vi "te_20200903.vi"() -> ()   [LabVIEW 2018]
uses:
  TE_ControlType_Enum.ctl
  TE_Polarity_Enum.ctl
  te_state.ctl
  TE_Main_Clust.ctl
  TE_Serial_Config_Clust.ctl
  Epimedia_Connex_Source/Controls/Clusts/TE_Data_Clust.ctl
  Epimedia_Connex_Source/Controls/Enums/WatchdogTimer_Enum.ctl
  Epimedia_Connex_Source/Controls/Enums/LogLoopEnum.ctl
  Disdrometer/UserConfig_ChannelSettings_Clust.ctl
panel:
  out "Shutdown if Alarm 3":bool
  out "Shutdown if Alarm 2":bool
  out "Shutdown if Alarm":bool
  out "LoAlarm3":dbl format="%.2g"
  out "LoAlarm2":dbl format="%.2g"
  out "LoAlarm":dbl format="%.2g"
  out "HiAlarm3":dbl format="%.2g"
  out "HiAlarm2":dbl format="%.2g"
  out "HiAlarm":dbl format="%.2g"
  out "Alarms? 3":bool
  out "Alarms? 2":bool
  out "Alarms?":bool
  in  "Shutdown if Alarm":bool=TRUE
  in  "Low Alarm":dbl=30.0 format="%.2g"
  in  "High Alarm":dbl=50.0 format="%.2g"
  in  "Alarms?":bool=TRUE
  out "AlarmStatus 3":T1(ring)
  out "AlarmStatus 2":T1(ring)
  out "AlarmStatus":T1(ring)
  out "On? 3":bool
  out "On? 2":bool
  in  "WriteFront":bool
  in  "WriteBottom":bool
  out "Polarity 3":T2
  out "Control Type 3":T3
  out "P 3":dbl format="%.2g"
  out "I 3":dbl format="%.2g"
  out "D 3":dbl format="%.2g"
  out "Set Point 3":dbl format="%.2g"
  out "Temp 3":dbl format="%.2g"
  out "Output 3":dbl format="%.2f"
  out "Polarity 2":T2
  out "Control Type 2":T3
  out "P 2":dbl format="%.2g"
  out "I 2":dbl format="%.2g"
  out "D 2":dbl format="%.2g"
  out "Set Point 2":dbl format="%.2g"
  out "Temp 2":dbl format="%.2g"
  out "Output 2":dbl format="%.2f"
  out "Polarity 4":T2
  in  "Polarity":T2 caption="Polarity*"
  out "Control Type 4":T3
  in  "Control Type":T3=enum."PID"
  in  "WriteAir":bool
  out "status":bool
  out "code":i32
  out "Read Progress":dbl(slide) scale=0.0..1.0
  out "On?":bool
  out "P 4":dbl format="%.2g"
  out "I 4":dbl format="%.2g"
  out "D 4":dbl format="%.2g"
  out "Set Point 4":dbl format="%.2g"
  out "Temp":dbl format="%.2g"
  out "Output":dbl format="%.2f"
  in  "On?":bool=TRUE
  in  "P":dbl=5.0 format="%.2g"
  in  "I":dbl format="%.2g"
  in  "D":dbl format="%.2g"
  in  "Set Point":dbl=40.0 format="%.2g"
  out "Header":picture
  in  "Address":string[](array[string])=["01", "02", "03"]
  in  "Port":refnum<visa-resource-name>="Port1"
  in  "stop":bool
  out "Error Dialog":string="Error Message Display Box"
  out "Waveform Chart":cluster{"[0]":dbl, "[0]":dbl, "[0]":dbl}(graph)
  # "°C"
  # "Temp."
  # "%"
  # "Output"
  # "°C"
  # "*Normal Polarity is WP1+ and WP2-\n  Reverse polarity is WP2+ and WP1-"
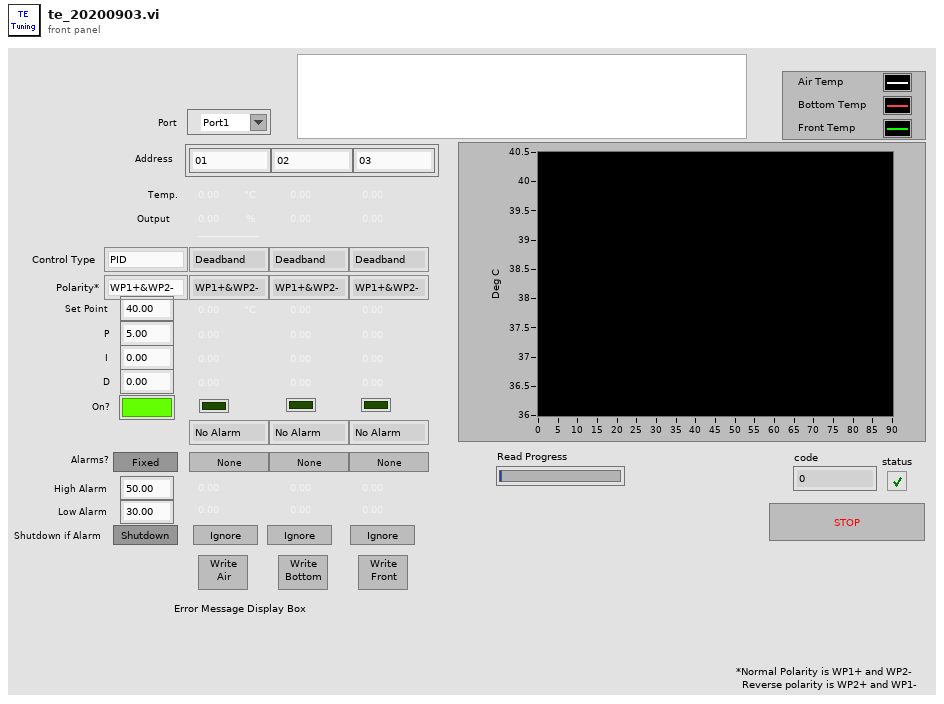
[diagram p1: front panel]
types:
  T1 = enum16{"No Alarm", "High Alarm", "Low Alarm", "Both Alarms"}
  T2 = typedef "TE_Polarity_Enum.ctl" = enum16{"WP1+&WP2-", "WP2+&WP1-"}
  T3 = typedef "TE_ControlType_Enum.ctl" = enum16{"Deadband", "PID", "Computer"}
  T4 = typedef "TE_Main_Clust.ctl" = cluster{"Serial":T5, "AcqData":dbl[][], "AcqSorted":T6, "WriteChannel":i32, "ErrMsg":string}
  T5 = typedef "TE_Serial_Config_Clust.ctl" = cluster{"port":refnum<visa-resource-name>, "timeout":u32, "baud":u32, "dataBits":u16, "stopBits":u16, "flowControl":u16, "parity":u16, "termChar":bool, "checkSum":bool, "checkSumVal":string, "Address":string[]}
  T6 = typedef "TE_Data_Clust.ctl" = cluster{"TimeString":string, "TimeStamp":dbl, "Temp":dbl, "Output":dbl, "Temp 2":dbl, "Output 2":dbl, "Temp 3":dbl, "Output 3":dbl}
  T7 = typedef "te_state.ctl" = enum16{"TE_Init", "TE_Autotune", "TE_Wait", "TE_Read", "TE_Display", "TE_Send", "TE_Write"}
  T8 = typedef "WatchdogTimer_Enum.ctl" = enum16{"ResetAll", "CheckAll", "HW1", "HW2", "Tones", "FP", "Noise", "Log", "TCP", "AI", "TC", "ADAM", "Disdrom", "TE", "Weather"}
  T9 = typedef "LogLoopEnum.ctl" = enum16{"Log_Init", "Log_Config", "Log_CfgAlarm", "Log_TimeDomain", "Log_Tone", "Log_NoiseTrace", "Log_NoiseSum", "Log_DO", "Log_AI", "Log_TC", "Log_Disdrom", "Log_Weather", "Log_TE", "Log_ADAM", "Log_UPS", "Log_ChkTime", "Log_Alarm", "Log_SSH", "Log_Write", "Log_Exit"}
  T10 = typedef "UserConfig_ChannelSettings_Clust.ctl" = cluster{"Set Point":dbl, "Control Type":T3, "Polarity":T2, "P":dbl, "I":dbl, "D":dbl, "On?":bool, "Alarms?":bool, "High Alarm":dbl, "Low Alarm":dbl, "Shutdown if Alarm":bool}
  T11 = typedef "imagedata.ctl" = cluster{"image type":i32, "image depth":i32, "image":u8[], "mask":u8[], "colors":u32[], "Rectangle":cluster{"left":i16, "top":i16, "right":i16, "bottom":i16}}
  T12 = cluster{"AcqData[0]":dbl, "AcqData[1]":dbl, "AcqData[2]":dbl, "AcqData[3]":dbl, "AcqData[4]":dbl, "AcqData[5]":dbl, "AcqData[6]":dbl, "AcqData[7]":dbl, "AcqData[8]":dbl, "AcqData[9]":dbl, "AcqData[10]":dbl, "AcqData[11]":dbl, "AcqData[12]":dbl, "AcqData[13]":dbl}
  T13 = cluster{"AcqData[0]":dbl, "AcqData[0]":dbl, "AcqData[0]":dbl}
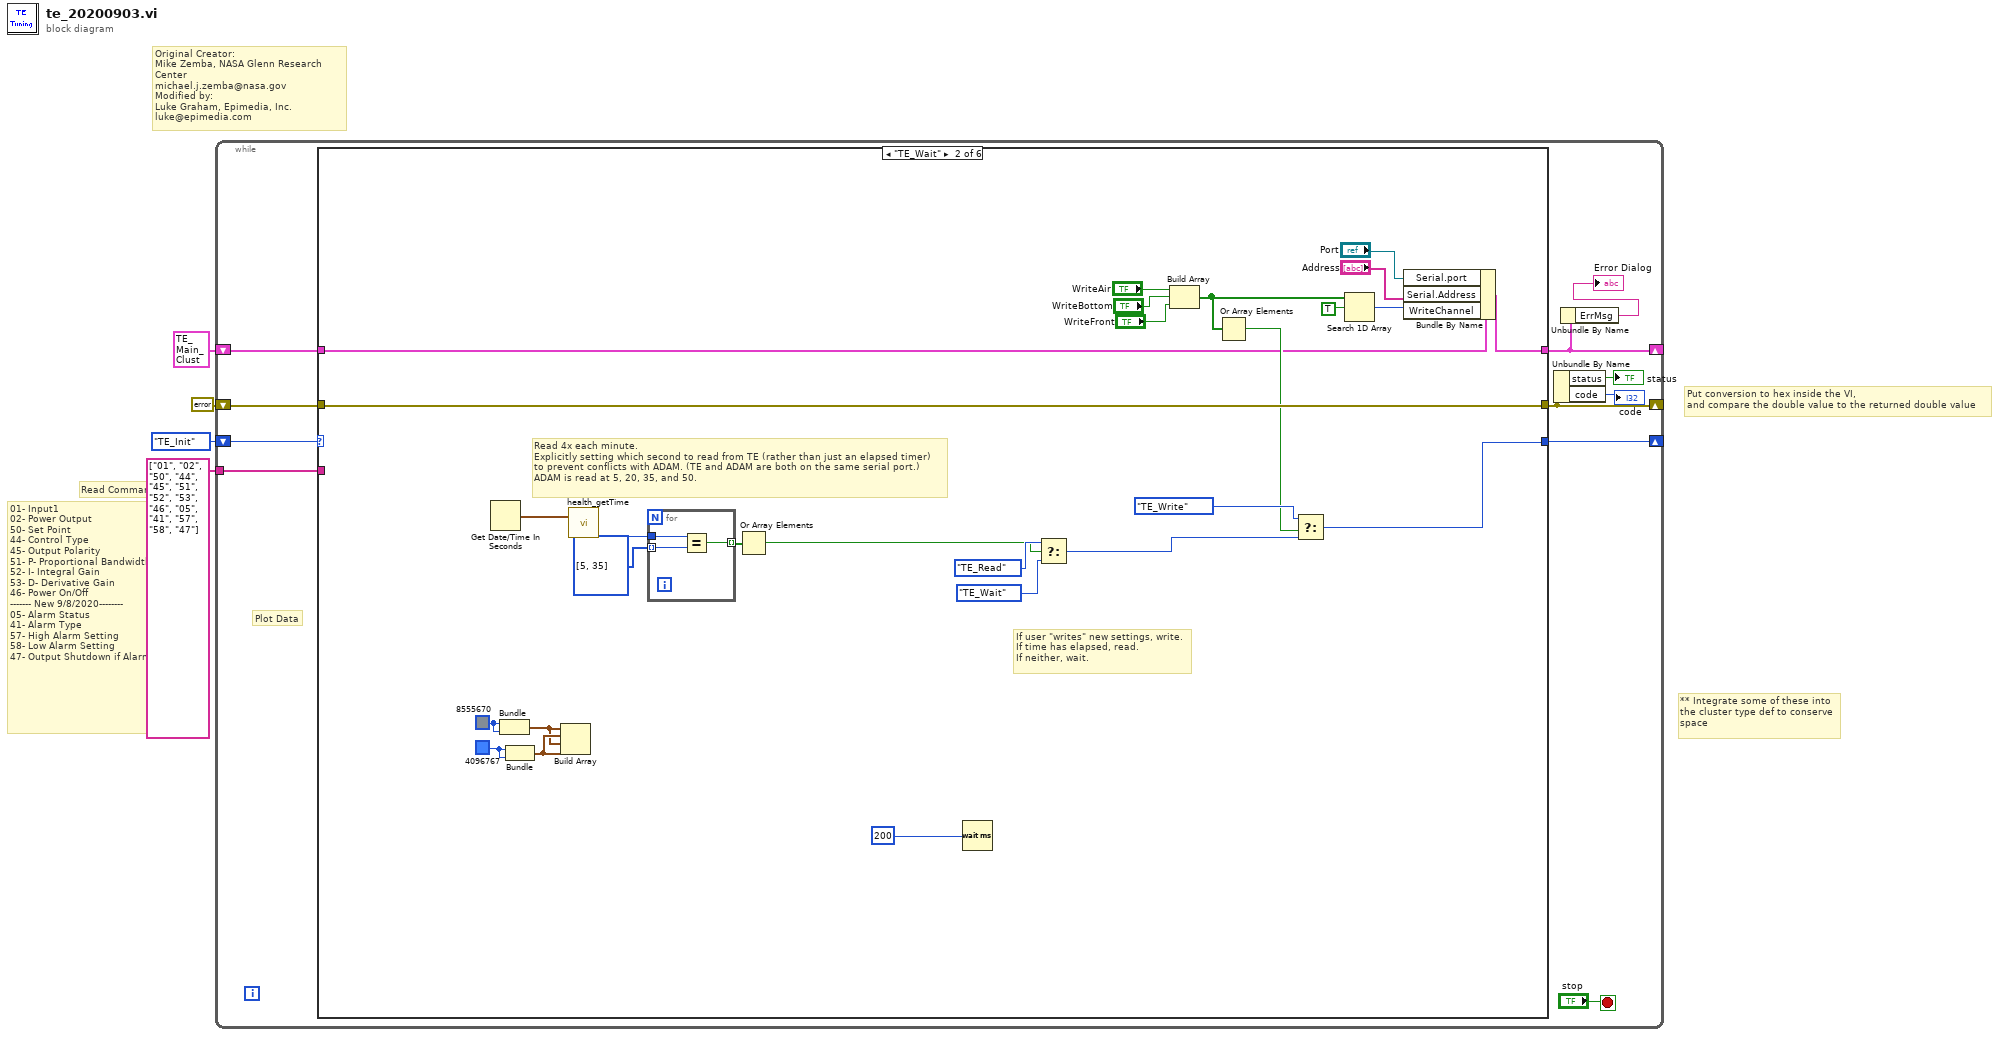
[diagram p0: block diagram]
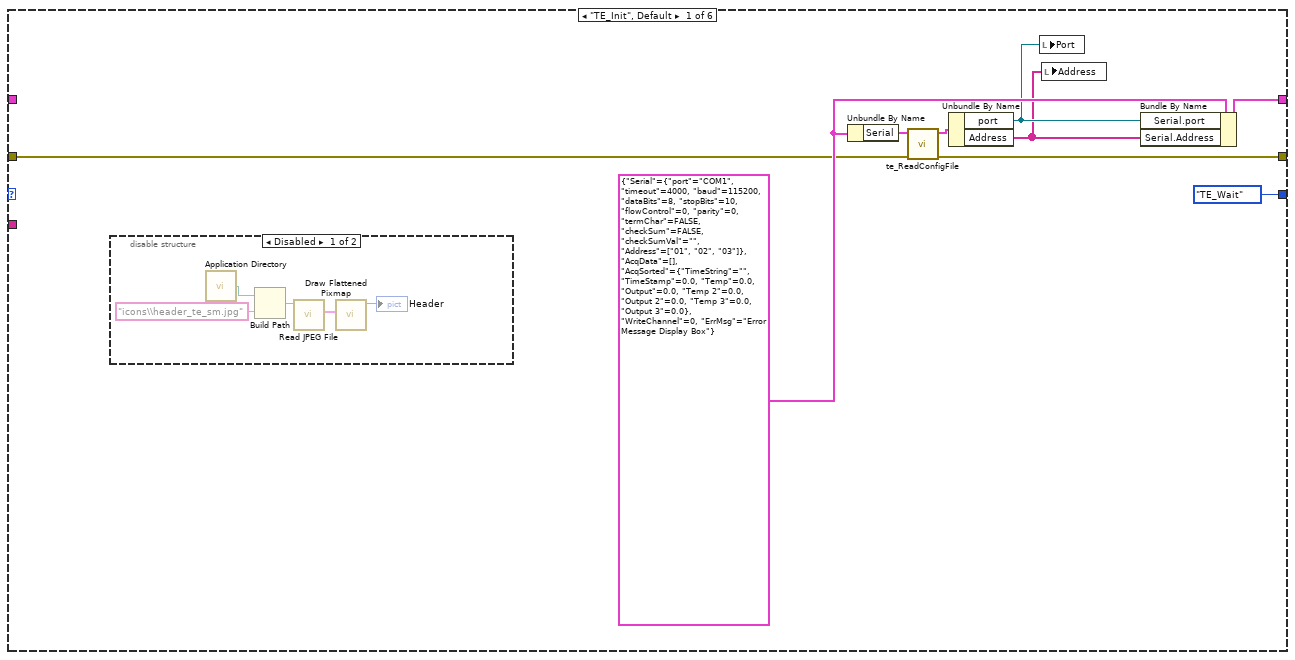
[diagram p2: hidden frame]
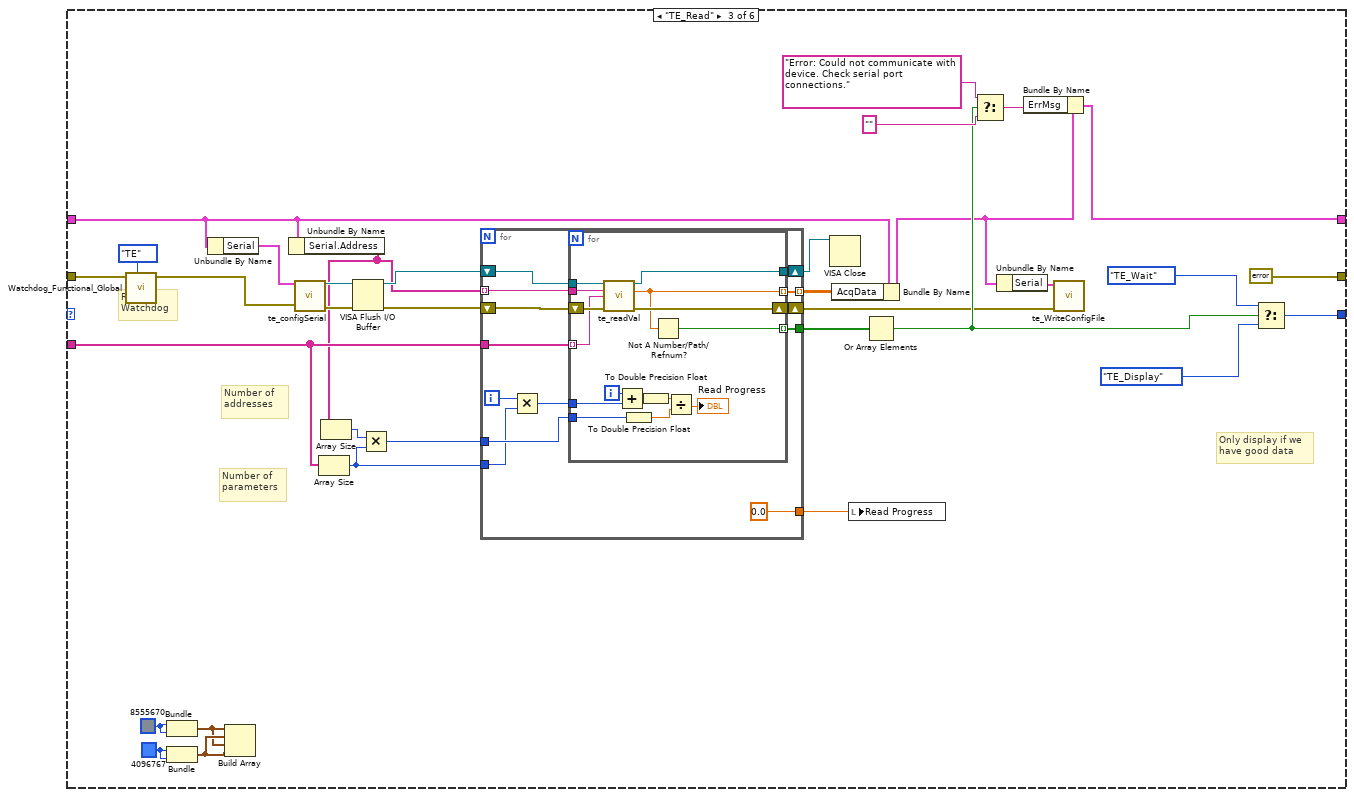
[diagram p4: hidden frame]
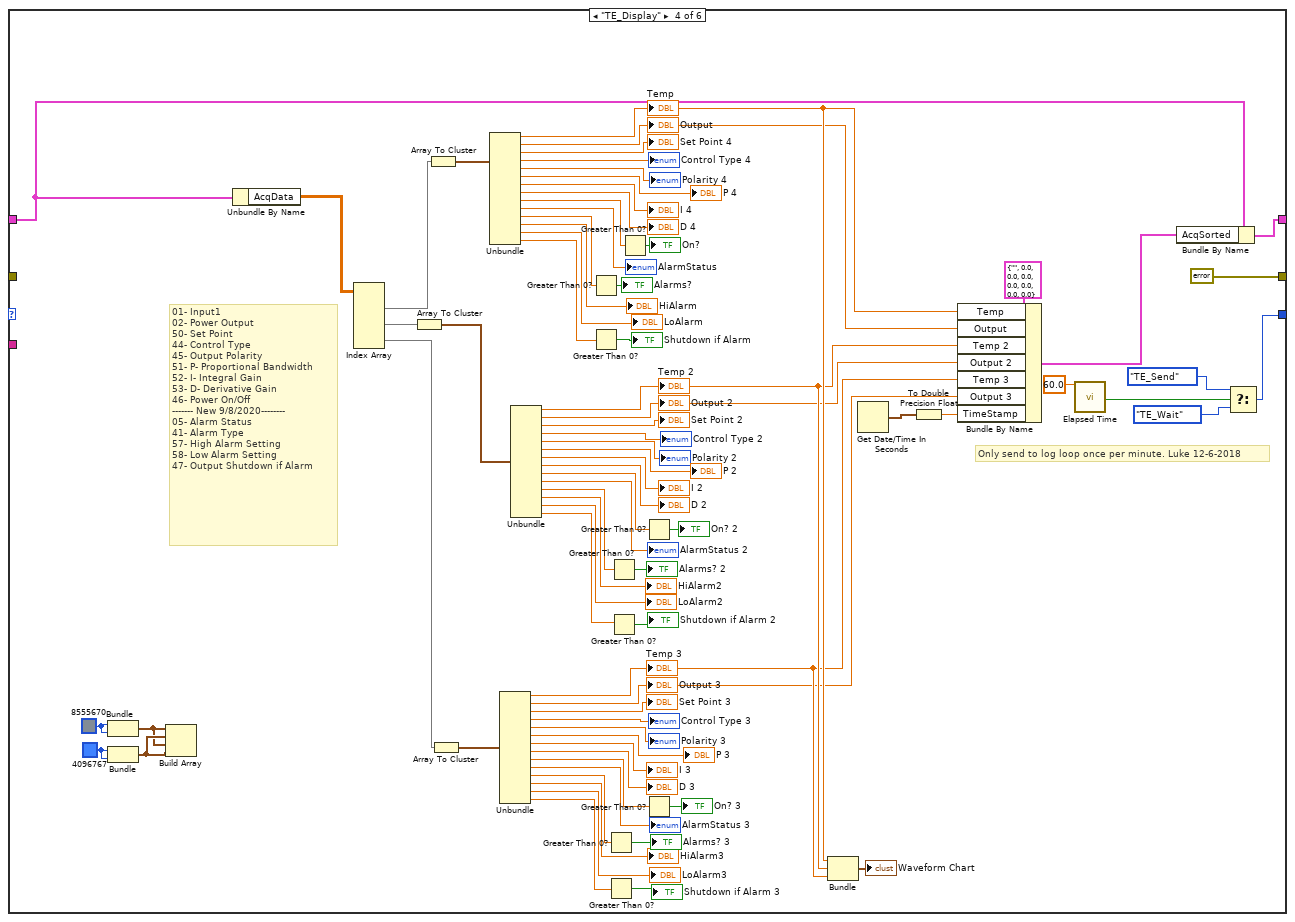
[diagram p5: hidden frame]
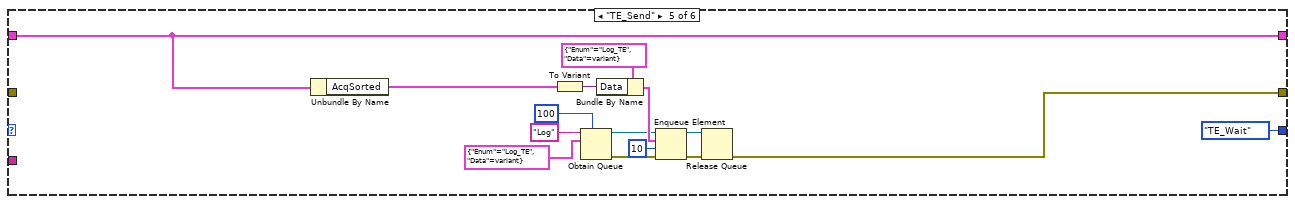
[diagram p6: hidden frame]
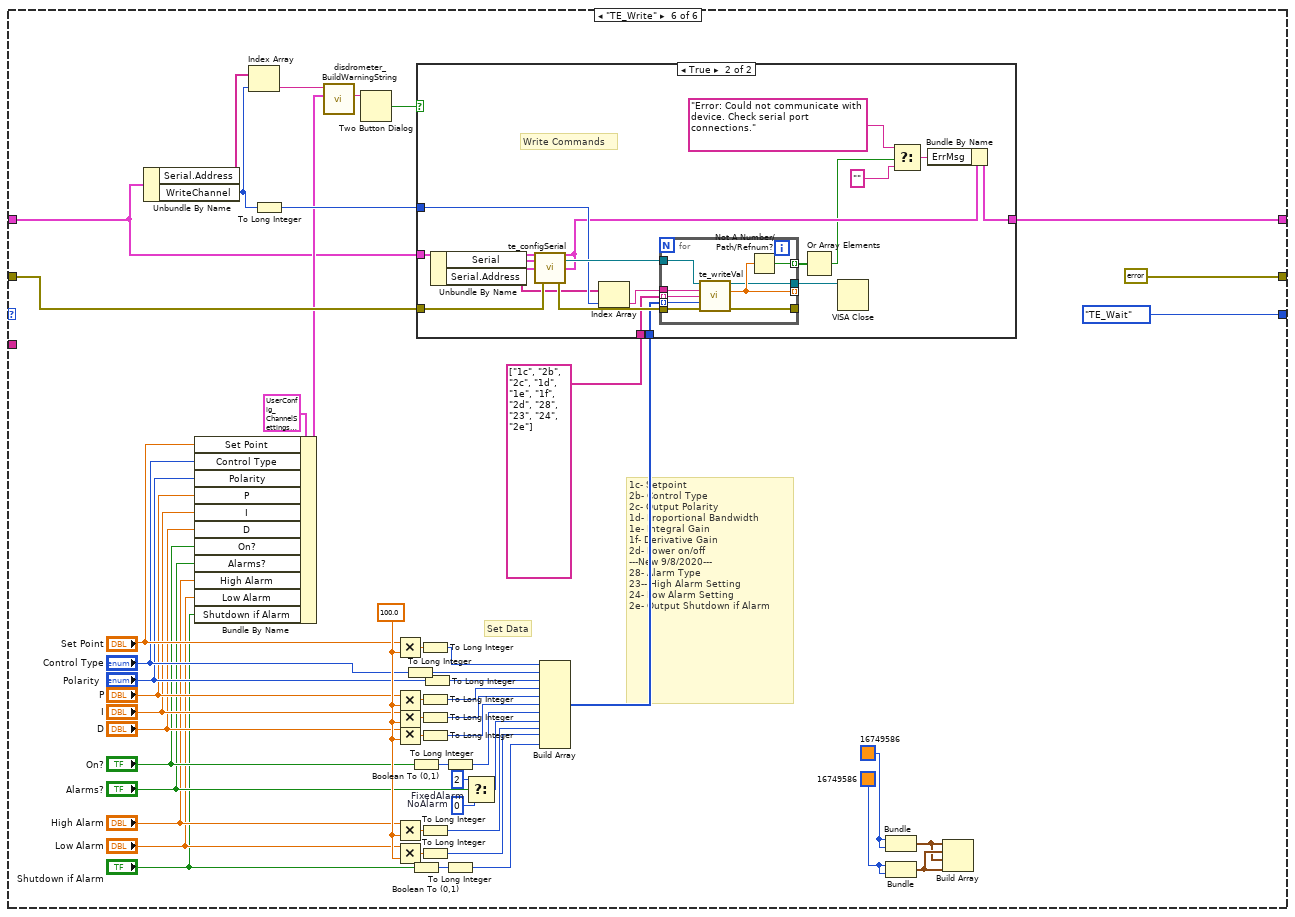
[diagram p7: hidden frame]
diagram:
  # "Original Creator: \nMike Zemba, NASA Glenn Research Center\nmichael.j.zemba@nasa.gov\nModified by:\nLuke Graham, Epimedia, Inc.\nluke@epimedia.com"
  # "Put conversion to hex inside the VI,\nand compare the double value to the returned double value"
  # "Read Commands"
  # "01- Input1\n02- Power Output\n50- Set Point\n44- Control Type\n45- Output Polarity\n51- P- Proportional Bandwidth\n52- I- Integral Gain\n53- D- Derivative Gain\n46- Power On/Off\n------- New 9/8/2020--------\n05- Alarm Status\n41- Alarm Type\n57- High Alarm Setting\n58- Low Alarm Setting\n47- Output Shutdown if Alarm"
  # "** Integrate some of these into\nthe cluster type def to conserve\nspace"
  n1 = while {
    shift-right: [w14] -> _
    shift-left: te_state."TE_Init" ("Enum") -> [w15]
    shift-right: [w9] -> _
    shift-left: errorcluster {"status"=FALSE, "code"=0, "source"=""} ("Error Out") -> [w13]
    tunnel: string[] ["01", "02", "50", "44", "45", "51", "52", "53", "46", "05", "41", "57", "58", "47"] -> [w10]
    shift-right: [w6] -> _
    shift-left: T4 {"Serial"={"port"="COM1", "timeout"=4000, "baud"=115200, "dataBits"=8, "stopBits"=10, "flowControl"=0, "parity"=0, "termChar"=FALSE, "checkSum"=FALSE, "checkSumVal"="", "Address"=["01", "02", "03"]}, "AcqData"=[], "AcqSorted"={"TimeString"="", "TimeStamp"=0.0, "Temp"=0.0, "Output"=0.0, "Temp 2"=0.0, "Output 2"=0.0, "Temp 3"=0.0, "Output 3"=0.0}, "WriteChannel"=0, "ErrMsg"="Error Message Display Box"} -> [w11]
    stop <- "stop" stop-if-true
    # "Plot Data"
    n2 = case shown="\"TE_Wait\"" w15 {
      tunnel: [te_state."TE_Wait" ("Enum") w46 w72 w161 te_state."TE_Wait" ("Enum") te_state."TE_Wait" ("Enum")] -> w14
      tunnel: w13 -> [w20 w52 w61 _ _ w257]
      tunnel: [w21 w52 errorcluster {"status"=FALSE, "code"=0, "source"=""} ("Error Out") errorcluster {"status"=FALSE, "code"=0, "source"=""} ("Error Out") w197 errorcluster {"status"=FALSE, "code"=0, "source"=""} ("Error Out")] -> w9
      tunnel: w11 -> [_ w33 w74 w164 w207 w217]
      tunnel: w10 -> [_ _ w82 _ _ _]
      tunnel: [w19 w34 w68 w165 w207 w218] -> w6
      frame "TE_Init", Default {
        w23 = T4 {"Serial"={"port"="COM1", "timeout"=4000, "baud"=115200, "dataBits"=8, "stopBits"=10, "flowControl"=0, "parity"=0, "termChar"=FALSE, "checkSum"=FALSE, "checkSumVal"="", "Address"=["01", "02", "03"]}, "AcqData"=[], "AcqSorted"={"TimeString"="", "TimeStamp"=0.0, "Temp"=0.0, "Output"=0.0, "Temp 2"=0.0, "Output 2"=0.0, "Temp 3"=0.0, "Output 3"=0.0}, "WriteChannel"=0, "ErrMsg"="Error Message Display Box"}
        n3 = disable-structure shown="Disabled" {
          frame Disabled {
            n4 = call <vilib>:"Application Directory.vi"() -> ("Application Directory"=w26:path)
            n5 = Build Path(base path=w26, name or relative path="icons\\header_te_sm.jpg") -> (appended path=w27:path)
            n6 = call <vilib>:"Read JPEG File.vi"("path to JPEG file"=w27) -> ("image data"=w29:T11)  [unwired: 8 in, 2 out]
            n7 = call <vilib>:"Draw Flattened Pixmap.vi"("image data"=w29) -> ("new picture"=→"Header":picture)  [unwired: 8 in]
          }
          frame Enabled {
          }
        }
        n8 = Unbundle By Name(w23) -> ("Serial"=w22:T5)
        n9 = call "te_ReadConfigFile.vi"("ErrorIn"=w20, "Serial"=w22) -> ("ErrorOut"=w21:errorcluster, "Serial"=w18:T5)  [unwired: 7 in, 1 out]
        n10 = Unbundle By Name(w18) -> ("port"=w17:refnum<visa-resource-name>, "Address"=w16:string[])
        n11 = local write "Port"(w17) -> ()
        n12 = local write "Address"(w16) -> ()
        n13 = Bundle By Name(cluster=w23, "Serial.port"=w17, "Serial.Address"=w16) -> (w19:T4)
      }
      frame "TE_Wait" {
        w56 = u32 4096767
        w55 = u32 8555670
        # "If user \"writes\" new settings, write.\nIf time has elapsed, read.\nIf neither, wait."
        # "Read 4x each minute.\nExplicitly setting which second to read from TE (rather than just an elapsed timer)\nto prevent conflicts with ADAM. (TE and ADAM are both on the same serial port.)\nADAM is read at 5, 20, 35, and 50."
        n14 = Get Date/Time In Seconds() -> (seconds since 1Jan1904=w41:timestamp)
        n15 = Bundle(w55, w55) -> (w53:cluster{u32, u32})  [unwired: 1 in]
        n16 = Bundle(w56, w56) -> (w54:cluster{u32, u32})  [unwired: 1 in]
        n17 = Build Array(w53, w54, w53, w54) -> ()  [unwired: 1 out]
        n18 = call "health_getTime.vi"("Current Time"=w41) -> ("Seconds"=w45:u32)  [unwired: 11 in, 7 out]
        n19 = for {
          tunnel: w45 -> [w59]
          tunnel: u32[] [5, 35] ("y") -> [w58] mode=indexing
          tunnel: [w57] -> w43 mode=indexing
          n20 = Equal?(x=w59, y=w58) -> (x = y?=w57:bool)
        }
        n21 = Or Array Elements(Boolean array=w43) -> (logical OR=w42:bool)
        n22 = Wait (ms)(milliseconds to wait=u32 200 ("y")) -> ()  [unwired: 1 out]
        n23 = Select(t=te_state."TE_Read" ("Enum"), s=w42, f=te_state."TE_Wait" ("Enum")) -> (s? t:f=w48:T7)
        n24 = Build Array("WriteAir", "WriteBottom", "WriteFront") -> (w36:bool[])
        n25 = Or Array Elements(Boolean array=w36) -> (logical OR=w35:bool)
        n26 = Select(t=te_state."TE_Write" ("Enum"), s=w35, f=w48) -> (s? t:f=w46:T7)
        n27 = Search 1D Array(1D array=w36, element=TRUE) -> (index of element=w32:i32)  [unwired: 1 in]
        n28 = Bundle By Name(cluster=w33, "Serial.port"="Port", "Serial.Address"="Address", "WriteChannel"=w32) -> (w34:T4)
      }
      frame "TE_Read" {
        w93 = u32 4096767
        w92 = u32 8555670
        # "Reset\nWatchdog"
        # "Only display if we\nhave good data"
        # "Number of parameters"
        # "Number of addresses"
        n29 = call "Watchdog_Functional_Global.vi"("Watchdog"=WatchdogTimer_Enum."TE", "error in"=w61) -> ("error out"=w60:errorcluster)  [unwired: 7 in, 2 out]
        n30 = Bundle(w92, w92) -> (w90:cluster{u32, u32})  [unwired: 1 in]
        n31 = Bundle(w93, w93) -> (w91:cluster{u32, u32})  [unwired: 1 in]
        n32 = Unbundle By Name(w74) -> ("Serial"=w75:T5)
        n33 = Build Array(w90, w91, w90, w91) -> ()  [unwired: 1 out]
        n34 = Unbundle By Name(w74) -> ("Serial.Address"=w73:string[])
        n35 = call "te_configSerial.vi"("Error In"=w60, "teSerial"=w75) -> ("error out"=w84:errorcluster, "VISA resource name out"=w86:refnum<visa-resource-name>)
        n36 = Array Size(array=w82) -> (size(s)=w79:i32)
        n37 = Array Size(array=w73) -> (size(s)=w80:i32)
        n38 = VISA Flush I/O Buffer(VISA resource name=w86, error in (no error)=w84) -> (VISA resource name out=w85:refnum<visa-resource-name>, error out=w83:errorcluster)  [unwired: 1 in]
        n39 = Multiply(x=w80, y=w79) -> (x*y=w81:i32)
        n40 = for {
          tunnel: [w106] -> w89
          tunnel: w82 -> [w105]
          tunnel: [w104] -> w78 mode=indexing
          tunnel: w73 -> [w101] mode=indexing
          shift-right: [w103] -> w87
          shift-left: w85 -> [w96]
          tunnel: w81 -> [w99]
          tunnel: w79 -> [w97]
          tunnel: [0.0 ("Read Progress")] -> w66
          shift-right: [w94] -> w65
          shift-left: w83 -> [w102]
          i -> [w100]
          n41 = Multiply(x=w100, y=w97) -> (x*y=w98:i32)
          n42 = for {
            tunnel: [w116] -> w104 mode=indexing
            tunnel: [w120] -> w106 mode=indexing
            tunnel: w101 -> [w118]
            tunnel: w105 -> [w117] mode=indexing
            tunnel: w96 -> [w115]
            tunnel: [w114] -> w103
            tunnel: w98 -> [w110]
            tunnel: w99 -> [w109]
            shift-right: [w119] -> w94
            shift-left: w102 -> [w121]
            i -> [w113]
            n43 = call "te_readVal.vi"("VISA In"=w115, "Hex Address"=w118, "Command"=w117, "Error In"=w121) -> ("VISA Out"=w114:refnum<visa-resource-name>, "Response"=w116:dbl, "error out"=w119:errorcluster)  [unwired: 7 in, 2 out]
            n44 = Add(x=w113, y=w110) -> (x+y=w112:i32)
            n45 = To Double Precision Float(number=w109) -> (double precision float=w107:dbl)
            n46 = To Double Precision Float(number=w112) -> (double precision float=w108:dbl)
            n47 = Not A Number/Path/Refnum?(number/path/refnum=w116) -> (NaN/Path/Refnum?=w120:bool)
            n48 = Divide(x=w108, y=w107) -> (x/y=→"Read Progress":dbl)
          }
        }
        n49 = VISA Close(VISA resource name=w87) -> ()  [unwired: 1 in, 1 out]
        n50 = Bundle By Name(cluster=w74, "AcqData"=w78) -> (w64:T4)
        n51 = local write "Read Progress"(w66) -> ()
        n52 = Or Array Elements(Boolean array=w89) -> (logical OR=w69:bool)
        n53 = Select(t="Error: Could not communicate with device. Check serial port connections." ("Error Dialog"), s=w69, f="" ("Error Dialog")) -> (s? t:f=w67:string)
        n54 = Unbundle By Name(w64) -> ("Serial"=w63:T5)
        n55 = Bundle By Name(cluster=w64, "ErrMsg"=w67) -> (w68:T4)
        n56 = call "te_WriteConfigFile.vi"("ErrorIn"=w65, "Serial"=w63) -> ()  [unwired: 9 in, 1 out]
        n57 = Select(t=te_state."TE_Wait", s=w69, f=te_state."TE_Display" ("Enum")) -> (s? t:f=w72:T7)
      }
      frame "TE_Display" {
        w196 = u32 4096767
        w195 = u32 8555670
        # "01- Input1\n02- Power Output\n50- Set Point\n44- Control Type\n45- Output Polarity\n51- P- Proportional Bandwidth\n52- I- Integral Gain\n53- D- Derivative Gain\n46- Power On/Off\n------- New 9/8/2020--------\n05- Alarm Status\n41- Alarm Type\n57- High Alarm Setting\n58- Low Alarm Setting\n47- Output Shutdown if Alarm"
        # "Only send to log loop once per minute. Luke 12-6-2018"
        n58 = Bundle(w195, w195) -> (w193:cluster{u32, u32})  [unwired: 1 in]
        n59 = Bundle(w196, w196) -> (w194:cluster{u32, u32})  [unwired: 1 in]
        n60 = Build Array(w193, w194, w193, w194) -> ()  [unwired: 1 out]
        n61 = Unbundle By Name(w164) -> ("AcqData"=w167:dbl[][])
        n62 = Index Array(array=w167) -> (element #1=w186:dbl[], element #2=w177:dbl[], element #3=w176:dbl[])  [unwired: 6 in]
        n63 = Array To Cluster(array=w177) -> (cluster=w185:T12)
        n64 = Array To Cluster(array=w186) -> (cluster=w191:T12)
        n65 = Array To Cluster(array=w176) -> (cluster=w178:T12)
        n66 = Unbundle(w191) -> ("AcqData[0]"=w173:dbl, "AcqData[1]"=w168:dbl, "AcqData[2]"=→"Set Point 4":dbl, "AcqData[3]"=→"Control Type 4":dbl, "AcqData[4]"=→"Polarity 4":dbl, "AcqData[5]"=→"P 4":dbl, "AcqData[6]"=→"I 4":dbl, "AcqData[7]"=→"D 4":dbl, "AcqData[8]"=w175:dbl, "AcqData[9]"=→"AlarmStatus":dbl, "AcqData[10]"=w142:dbl, "AcqData[11]"=→"HiAlarm":dbl, "AcqData[12]"=→"LoAlarm":dbl, "AcqData[13]"=w132:dbl)
        "Temp" <- w173
        "Output" <- w168
        n67 = Unbundle(w178) -> ("AcqData[0]"=w171:dbl, "AcqData[1]"=w170:dbl, "AcqData[2]"=→"Set Point 3":dbl, "AcqData[3]"=→"Control Type 3":dbl, "AcqData[4]"=→"Polarity 3":dbl, "AcqData[5]"=→"P 3":dbl, "AcqData[6]"=→"I 3":dbl, "AcqData[7]"=→"D 3":dbl, "AcqData[8]"=w151:dbl, "AcqData[9]"=→"AlarmStatus 3":dbl, "AcqData[10]"=w144:dbl, "AcqData[11]"=→"HiAlarm3":dbl, "AcqData[12]"=→"LoAlarm3":dbl, "AcqData[13]"=w130:dbl)
        "Temp 3" <- w171
        "Output 3" <- w170
        n68 = Unbundle(w185) -> ("AcqData[0]"=w172:dbl, "AcqData[1]"=w169:dbl, "AcqData[2]"=→"Set Point 2":dbl, "AcqData[3]"=→"Control Type 2":dbl, "AcqData[4]"=→"Polarity 2":dbl, "AcqData[5]"=→"P 2":dbl, "AcqData[6]"=→"I 2":dbl, "AcqData[7]"=→"D 2":dbl, "AcqData[8]"=w150:dbl, "AcqData[9]"=→"AlarmStatus 2":dbl, "AcqData[10]"=w143:dbl, "AcqData[11]"=→"HiAlarm2":dbl, "AcqData[12]"=→"LoAlarm2":dbl, "AcqData[13]"=w128:dbl)
        "Temp 2" <- w172
        "Output 2" <- w169
        n69 = Greater Than 0?(x=w142) -> (x > 0?=→"Alarms?":bool)
        n70 = Greater Than 0?(x=w132) -> (x > 0?=→"Shutdown if Alarm":bool)
        n71 = Greater Than 0?(x=w144) -> (x > 0?=→"Alarms? 3":bool)
        n72 = Greater Than 0?(x=w130) -> (x > 0?=→"Shutdown if Alarm 3":bool)
        n73 = Greater Than 0?(x=w143) -> (x > 0?=→"Alarms? 2":bool)
        n74 = Greater Than 0?(x=w128) -> (x > 0?=→"Shutdown if Alarm 2":bool)
        n75 = Greater Than 0?(x=w175) -> (x > 0?=→"On?":bool)
        n76 = Greater Than 0?(x=w150) -> (x > 0?=→"On? 2":bool)
        n77 = Greater Than 0?(x=w151) -> (x > 0?=→"On? 3":bool)
        n78 = Bundle("AcqData[0]"=w173, "AcqData[0]"=w172, "AcqData[0]"=w171) -> (→"Waveform Chart":T13)  [unwired: 1 in]
        n79 = Get Date/Time In Seconds() -> (seconds since 1Jan1904=w122:timestamp)
        n80 = To Double Precision Float(number=w122) -> (double precision float=w123:dbl)
        n81 = Bundle By Name(cluster=T6 {"TimeString"="", "TimeStamp"=0.0, "Temp"=0.0, "Output"=0.0, "Temp 2"=0.0, "Output 2"=0.0, "Temp 3"=0.0, "Output 3"=0.0}, "Temp"=w173, "Output"=w168, "Temp 2"=w172, "Output 2"=w169, "Temp 3"=w171, "Output 3"=w170, "TimeStamp"=w123) -> (w163:T6)
        n82 = call "Elapsed Time"("Time Target (s)"=60.0) -> ("Time has Elapsed"=w160:bool)  [unwired: 11 in, 7 out]
        n83 = Bundle By Name(cluster=w164, "AcqSorted"=w163) -> (w165:T4)
        n84 = Select(t=te_state."TE_Send", s=w160, f=te_state."TE_Wait" ("Enum")) -> (s? t:f=w161:T7)
      }
      frame "TE_Send" {
        n85 = Unbundle By Name(w207) -> ("AcqSorted"=w208:T6)
        n86 = To Variant(anything=w208) -> (Variant=w209:variant)
        n87 = Obtain Queue(max queue size (-1, unlimited)=100, name (unnamed)="Log", element data type=cluster{"Enum":T9, "Data":variant} {"Enum"=enum."Log_TE", "Data"=variant}) -> (queue out=w201:refnum<queue>, error out=w202:errorcluster)  [unwired: 2 in, 1 out]
        n88 = Bundle By Name(cluster=cluster{"Enum":T9, "Data":variant} {"Enum"=enum."Log_TE", "Data"=variant}, "Data"=w209) -> (w211:cluster{"Enum":T9, "Data":variant})
        n89 = Enqueue Element(queue=w201, element=w211, timeout in ms (-1)=10, error in (no error)=w202) -> (queue out=w203:refnum<queue>, error out=w204:errorcluster)  [unwired: 1 out]
        n90 = Release Queue(queue=w203, error in (no error)=w204) -> (error out=w197:errorcluster)  [unwired: 1 in, 2 out]
      }
      frame "TE_Write" {
        w240 = 0  # NoAlarm
        w241 = 2  # FixedAlarm
        w235 = 100.0 ("y")
        w262 = u32 16749586
        w261 = u32 16749586
        # "1c- Setpoint\n2b- Control Type\n2c- Output Polarity\n1d- Proportional Bandwidth\n1e- Integral Gain\n1f- Derivative Gain\n2d- Power on/off\n---New 9/8/2020---\n28- Alarm Type\n23-- High Alarm Setting\n24- Low Alarm Setting\n2e- Output Shutdown if Alarm"
        # "Set Data"
        n91 = Unbundle By Name(w217) -> ("Serial.Address"=w213:string[], "WriteChannel"=w214:i32)
        n92 = Bundle By Name(cluster=T10 {"Set Point"=40.0, "Control Type"=enum."Deadband", "Polarity"=enum."WP1+&WP2-", "P"=5.0, "I"=0.0, "D"=0.0, "On?"=FALSE, "Alarms?"=FALSE, "High Alarm"=0.0, "Low Alarm"=0.0, "Shutdown if Alarm"=FALSE} ("UserCfg"), "Set Point"="Set Point", "Control Type"="Control Type", "Polarity"="Polarity", "P"="P", "I"="I", "D"="D", "On?"="On?", "Alarms?"="Alarms?", "High Alarm"="High Alarm", "Low Alarm"="Low Alarm", "Shutdown if Alarm"="Shutdown if Alarm") -> (w219:T10)
        n93 = Index Array(array=w213, index=w214) -> (element=w212:string)
        n94 = To Long Integer(number=w214) -> (32bit integer=w246:i32)
        n95 = call "disdrometer_BuildWarningString.vi"("UserCfg"=w219, "WriteChannel"=w212) -> ("WarningString"=w216:string)  [unwired: 9 in]
        n96 = Two Button Dialog(message=w216) -> (T button?=w215:bool)  [unwired: 2 in]
        n97 = Multiply(x="Set Point", y=w235) -> (x*y=w248:dbl)
        n98 = Multiply(x="P", y=w235) -> (x*y=w251:dbl)
        n99 = Multiply(x="I", y=w235) -> (x*y=w250:dbl)
        n100 = Multiply(x="D", y=w235) -> (x*y=w249:dbl)
        n101 = Multiply(x="High Alarm", y=w235) -> (x*y=w238:dbl)
        n102 = Multiply(x="Low Alarm", y=w235) -> (x*y=w236:dbl)
        n103 = To Long Integer(number="Control Type") -> (32bit integer=w245:i32)
        n104 = Boolean To (0,1)(Boolean="On?") -> (0, 1=w243:i16)
        n105 = Boolean To (0,1)(Boolean="Shutdown if Alarm") -> (0, 1=w233:i16)
        n106 = To Long Integer(number=w248) -> (32bit integer=w252:i32)
        n107 = To Long Integer(number=w251) -> (32bit integer=w253:i32)
        n108 = To Long Integer(number=w250) -> (32bit integer=w254:i32)
        n109 = To Long Integer(number=w249) -> (32bit integer=w255:i32)
        n110 = To Long Integer(number=w238) -> (32bit integer=w237:i32)
        n111 = To Long Integer(number=w236) -> (32bit integer=w234:i32)
        n112 = To Long Integer(number="Polarity") -> (32bit integer=w244:i32)
        n113 = To Long Integer(number=w243) -> (32bit integer=w242:i32)
        n114 = To Long Integer(number=w233) -> (32bit integer=w232:i32)
        n115 = Select(t=w241, s="Alarms?", f=w240) -> (s? t:f=w239:i32)
        n116 = Build Array(w252, w245, w244, w253, w254, w255, w242, w239, w237, w234, w232) -> (w247:i32[])
        n117 = case shown="True" w215 {
          tunnel: w257 -> [_ w278]
          tunnel: string[] ["1c", "2b", "2c", "1d", "1e", "1f", "2d", "28", "23", "24", "2e"] -> [_ w276]
          tunnel: w247 -> [_ w275]
          tunnel: w246 -> [_ w273]
          tunnel: [w264 w270] -> w218
          tunnel: w217 -> [w264 w269]
          frame False {
          }
          frame True {
            # "Write Commands"
            n118 = Unbundle By Name(w269) -> ("Serial"=w272:T5, "Serial.Address"=w271:string[])
            n119 = call "te_configSerial.vi"("Error In"=w278, "teSerial"=w272) -> ("error out"=w279:errorcluster, "VISA resource name out"=w280:refnum<visa-resource-name>)
            n120 = Index Array(array=w271, index=w273) -> (element=w274:string)
            n121 = for {
              tunnel: [w285] -> _ mode=indexing
              tunnel: w279 -> [w290]
              tunnel: [w289] -> w281 mode=indexing
              tunnel: [w288] -> _
              tunnel: w274 -> [w287]
              tunnel: w276 -> [w286] mode=indexing
              tunnel: w280 -> [w284]
              tunnel: [w283] -> w277
              tunnel: w275 -> [w282] mode=indexing
              n122 = call "te_writeVal.vi"("VISA In"=w284, "Hex Address"=w287, "Command"=w286, "Data"=w282, "Error In"=w290) -> ("VISA Out"=w283:refnum<visa-resource-name>, "Response"=w285:dbl, "error out"=w288:errorcluster)  [unwired: 7 in, 1 out]
              n123 = Not A Number/Path/Refnum?(number/path/refnum=w285) -> (NaN/Path/Refnum?=w289:bool)
            }
            n124 = Or Array Elements(Boolean array=w281) -> (logical OR=w266:bool)
            n125 = VISA Close(VISA resource name=w277) -> ()  [unwired: 1 in, 1 out]
            n126 = Select(t="Error: Could not communicate with device. Check serial port connections." ("Error Dialog"), s=w266, f="" ("Error Dialog")) -> (s? t:f=w265:string)
            n127 = Bundle By Name(cluster=w269, "ErrMsg"=w265) -> (w270:T4)
          }
        }
        n128 = Bundle(w261, w261) -> (w259:cluster{u32, u32})  [unwired: 1 in]
        n129 = Bundle(w262, w262) -> (w260:cluster{u32, u32})  [unwired: 1 in]
        n130 = Build Array(w259, w260, w259, w260) -> ()  [unwired: 1 out]
      }
    }
    n131 = Unbundle By Name(w9) -> ("status"=→"status":bool, "code"=→"code":i32)
    n132 = Unbundle By Name(w6) -> ("ErrMsg"=→"Error Dialog":string)
  }
